vi "TSM SSC DCPower MeasureWhen.vi"(8 "error in":errorcluster, 10 "Measurement:Advanced:Measure When":i32(ring)=1025 items=["Automatically after Source Complete"=1025, "On Demand"=1026, "On Measure Trigger"=1027], 11 "DCPower SSC in":T1[](array[typedef])) -> (0 "error out":errorcluster, 3 "DCPower SSC out":T1[](array[typedef]))   [LabVIEW 2019]
uses:
  SSC DCPower/SSC DCPower.ctl
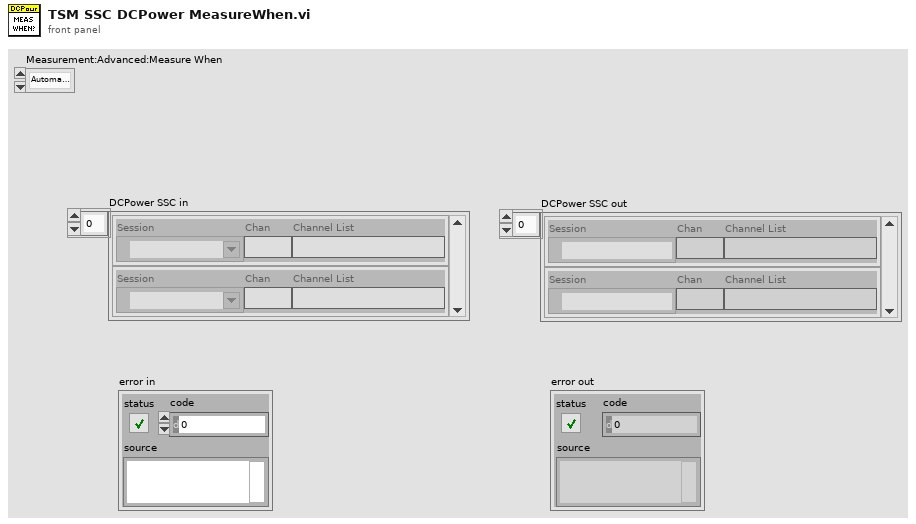
[diagram p1: front panel]
types:
  T1 = typedef "SSC DCPower.ctl" = cluster{"Session":refnum<k15>, "Chan":string, "Channel List":string}
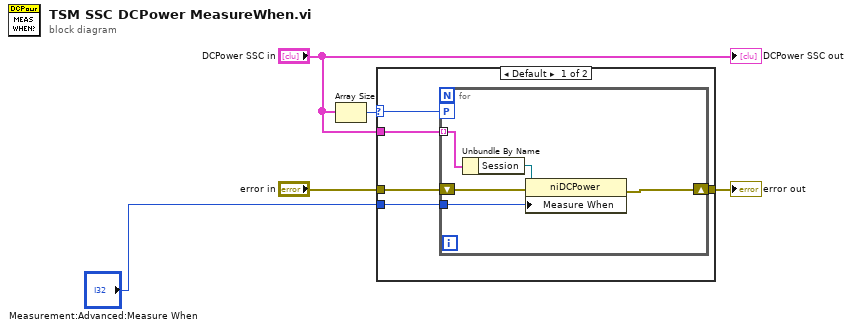
[diagram p0: block diagram]
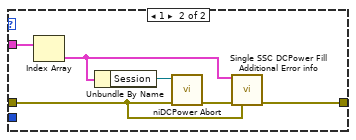
[diagram p2: hidden frame]
diagram:
  n1 = Array Size(array="DCPower SSC in") -> (size(s)=w3:i32)
  n2 = case shown="Default" w3 {
    selector: w3 -> [w8 _]
    tunnel: "error in" -> [w10 w21]
    tunnel: [w9 w20] -> w4
    tunnel: "DCPower SSC in" -> [w7 w19]
    tunnel: "Measurement:Advanced:Measure When" -> [w6 _]
    frame Default {
      n3 = for {
        tunnel: w7 -> [w15] mode=indexing
        workers-P: w8 -> [_]
        shift-right: [w12] -> w9
        shift-left: w10 -> [w13]
        tunnel: w6 -> [w11]
        n4 = Unbundle By Name(w15) -> ("Session"=w14:refnum<k15>)
        n5 = property class="niDCPower"(reference=w14, error in=w13, "Measure When"=w11) -> (error out=w12:errorcluster)  [unwired: 1 out]
      }
    }
    frame 1 {
      n6 = Index Array(array=w19) -> (element=w16:T1)  [unwired: 1 in]
      n7 = Unbundle By Name(w16) -> ("Session"=w17:refnum<k15>)
      n8 = call <instrlib>:"niDCPower Abort.vi"("error in (no error)"=w21, "instrument handle"=w17) -> ("error out"=w18:errorcluster)  [unwired: 8 in, 1 out]
      n9 = call "Single SSC DCPower Fill Additional Error info.vi"("DCPower SSC in"=w16, "error in"=w18, "previous error in"=w21) -> ("error out"=w20:errorcluster)  [unwired: 12 in]
    }
  }
  "error out" <- w4
  "DCPower SSC out" <- "DCPower SSC in"
